vi "Send move to stages.vi"(8 "error in (no error)":errorcluster, 11 "Tomo in":refnum<class "Tomo.lvclass">) -> (0 "error out":errorcluster, 3 "Tomo out":refnum<class "Tomo.lvclass">)   [LabVIEW 2012, in "Tomo.lvclass"]
uses:
  Tomo.lvclass
  <vilib>/Distrio/Murmex/GenericMessage/GenericMessage.lvclass
  <vilib>/Distrio/Murmex/StartMessage/StartMessage.lvclass
  <vilib>/Distrio/Murmex/Message/Message.lvclass
  <vilib>/Distrio/Murmex/Murmex/Murmex.lvclass
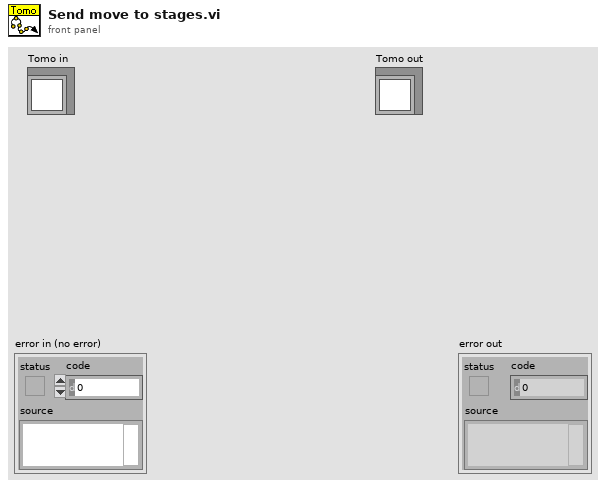
[diagram p1: front panel]
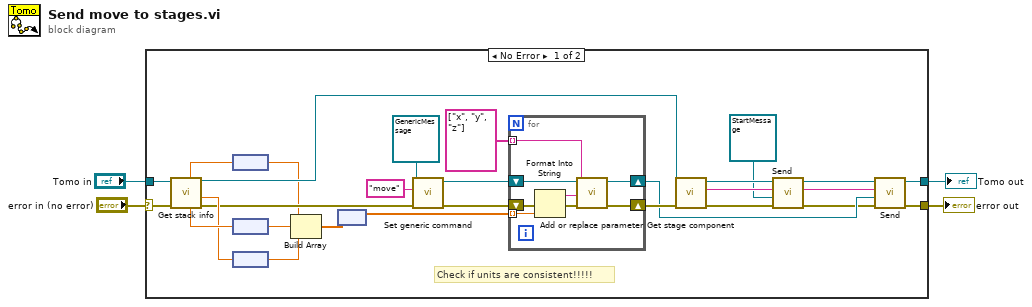
[diagram p0: block diagram]
diagram:
  n1 = case shown="No Error" "error in (no error)" {
    selector: "error in (no error)" -> [w28 w41]
    tunnel: [w19 w41] -> w3
    tunnel: [w20 w40] -> w2
    tunnel: "Tomo in" -> [w29 w40]
    frame No Error {
      # "Check if units are consistent!!!!!"
      n2 = call-dynamic "Get stack info.vi"("error in (no error)"=w28, "Tomo in"=w29) -> ("error out"=w15:errorcluster, "Z start"=w25:dbl, "Tomo out"=w14:refnum<class "Tomo.lvclass">, "Y position"=w26:dbl, "X position"=w27:dbl)  [unwired: 4 in, 1 out]
      n3 = node(w27) -> (w11:dbl[unit])
      n4 = node(w26) -> (w13:dbl[unit])
      n5 = node(w25) -> (w12:dbl[unit])
      n6 = Build Array(w11, w13, w12) -> (w21:dbl[unit][])
      n7 = node(w21) -> (w16:dbl[])
      n8 = call <vilib>:"Set generic command.vi"("error in (no error)"=w15, "generic command"="move" ("command string"), "GenericMessage in"=refnum<class "GenericMessage.lvclass"> refnum ("Murmex.lvlib:GenericMessage")) -> ("error out"=w24:errorcluster, "GenericMessage out"=w23:refnum<class "GenericMessage.lvclass">)  [unwired: 7 in]
      n9 = for {
        shift-right: [w33] -> w18
        shift-left: w24 -> [w39]
        shift-right: [w34] -> w17
        shift-left: w23 -> [w38]
        tunnel: string[] ["x", "y", "z"] -> [w36] mode=indexing
        tunnel: w16 -> [w35] mode=indexing
        n10 = Format Into String(error in=w39, w35) -> (resulting string=w32:string, error out=w37:errorcluster)  [unwired: 2 in]
        n11 = call <vilib>:"Add or replace parameter.vi"("error in (no error)"=w37, "value"=w32, "name"=w36, "Message in"=w38) -> ("error out"=w33:errorcluster, "Message out"=w34:refnum<class "GenericMessage.lvclass">)  [unwired: 6 in]
      }
      n12 = call-dynamic "Get stage component.vi"("error in (no error)"=w18, "Tomo in"=w14) -> ("error out"=w10:errorcluster, "stage component"=w6:string, "Tomo out"=w8:refnum<class "Tomo.lvclass">)  [unwired: 7 in]
      n13 = call <vilib>:"Send.vi"("error in (no error)"=w10, "Message"=refnum<class "StartMessage.lvclass"> refnum ("Distrio Murmex 1.1:StartMessage"), "recipient"=w6, "Murmex in"=w8) -> ("error out"=w9:errorcluster, "Murmex out"=w7:refnum<class "Tomo.lvclass">)  [unwired: 6 in]
      n14 = call <vilib>:"Send.vi"("error in (no error)"=w9, "Message"=w17, "recipient"=w6, "Murmex in"=w7) -> ("error out"=w19:errorcluster, "Murmex out"=w20:refnum<class "Tomo.lvclass">)  [unwired: 6 in]
    }
    frame Error {
    }
  }
  "error out" <- w3
  "Tomo out" <- w2
